vi "Read Print Options.vi"(8 "error in (no error)":errorcluster, 11 "WebView2 Control in":refnum<class "WebView2 Control.lvclass">) -> (0 "error out":errorcluster, 2 "CreatePrintSettings":refnum<k24>, 3 "WebView2 Control out":refnum<class "WebView2 Control.lvclass">)   [LabVIEW 2020, in "WebView2.lvlib" / "WebView2 Control.lvclass"]
uses:
  WebView2 Control.lvclass
  C:/Users/Simon/Documents/GitHub/LV-WebView2/Source/Libs/Microsoft.Web.WebView2.Core.dll
  Libs/Microsoft.Web.WebView2.Core.dll
  Read Environment.vi
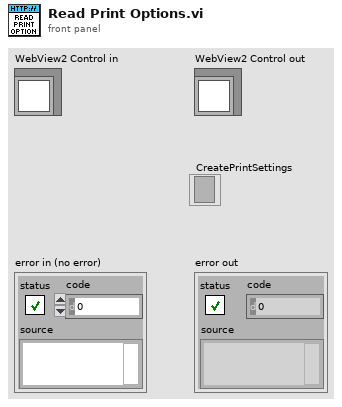
[diagram p1: front panel]
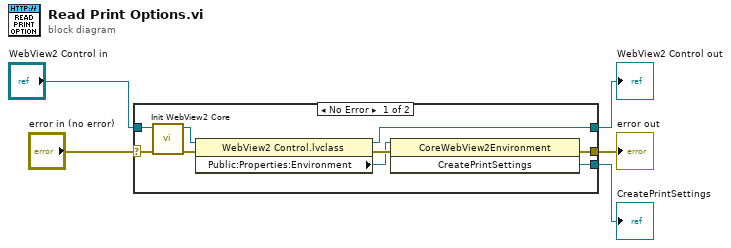
[diagram p0: block diagram]
diagram:
  n1 = case shown="No Error" "error in (no error)" {
    selector: "error in (no error)" -> [w13 w16]
    tunnel: [w11 w16] -> w4
    tunnel: [w7 w15] -> w2
    tunnel: "WebView2 Control in" -> [w14 w15]
    tunnel: [w10 _] -> w1
    frame No Error {
      n2 = call "Init WebView2 Core.vi"("error in (no error)"=w13, "WebView2"=w14) -> ("error out"=w12:errorcluster, "WebView2.lvlib:WebView2 Control.lvclass"=w8:refnum<class "WebView2 Control.lvclass">)  [unwired: 8 in]
      n3 = property class="WebView2 Control.lvclass"(reference=w8, error in=w12) -> (reference out=w7:refnum<class "WebView2 Control.lvclass">, error out=w9:errorcluster, "Public:Properties:Environment"=w6:refnum<k24>)
      n4 = invoke class="CoreWebView2Environment" method="CreatePrintSettings"(reference=w6, error in=w9) -> (error out=w11:errorcluster, "CreatePrintSettings"=w10:refnum<k24>)  [unwired: 1 in, 1 out]
    }
    frame Error {
    }
  }
  "error out" <- w4
  "WebView2 Control out" <- w2
  "CreatePrintSettings" <- w1
